vi "Json_Data_Path.vi"(8 "error in":errorcluster, 10 "ERD Data In":cluster{"ERD Number":u16, "Data":string}[](array[cluster]) {"ERD Number" format="%.0x"}, 11 "Json File Path":path) -> (0 "error out":errorcluster, 2 "ERD Data Out":cluster{"ERD Number":u16, "Data":string}[](array[cluster]) {"ERD Number" format="%.0x"})   [LabVIEW 2021]
uses:
  <vilib>/JDP Science/JSONtext/String Subset.vi
  <vilib>/JDP Science/JSONtext/support/Strip Quotes and Unescape.vi
  <vilib>/JDP Science/JSONtext/support/Unescape JSON string.vi
  <vilib>/JDP Science/JSONtext/Parsing/Parse Full Path or Item Name.vi
  <vilib>/JDP Science/JSONtext/Offset/Find Item Locations by Path.vi
  <vilib>/JDP Science/JSONtext/JSONtext.lvlib
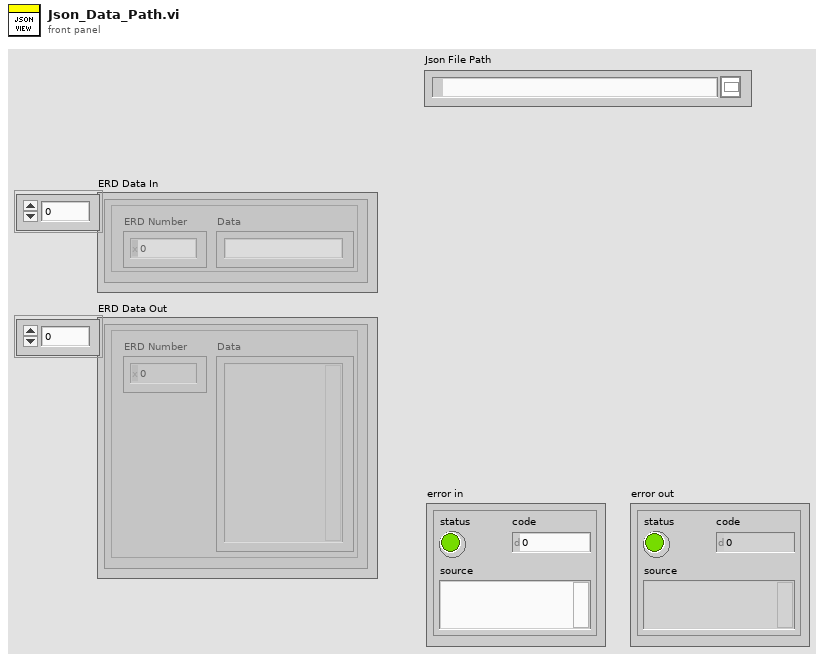
[diagram p1: front panel]
types:
  T1 = cluster{"ERD Data In[0]":cluster{"ERD Number":u16, "Data":string}, "ERD Data In[1]":cluster{"ERD Number":u16, "Data":string}, "ERD Data In[2]":cluster{"ERD Number":u16, "Data":string}, "ERD Data In[3]":cluster{"ERD Number":u16, "Data":string}, "ERD Data In[4]":cluster{"ERD Number":u16, "Data":string}, "ERD Data In[5]":cluster{"ERD Number":u16, "Data":string}, "ERD Data In[6]":cluster{"ERD Number":u16, "Data":string}, "ERD Data In[7]":cluster{"ERD Number":u16, "Data":string}, "ERD Data In[8]":cluster{"ERD Number":u16, "Data":string}}
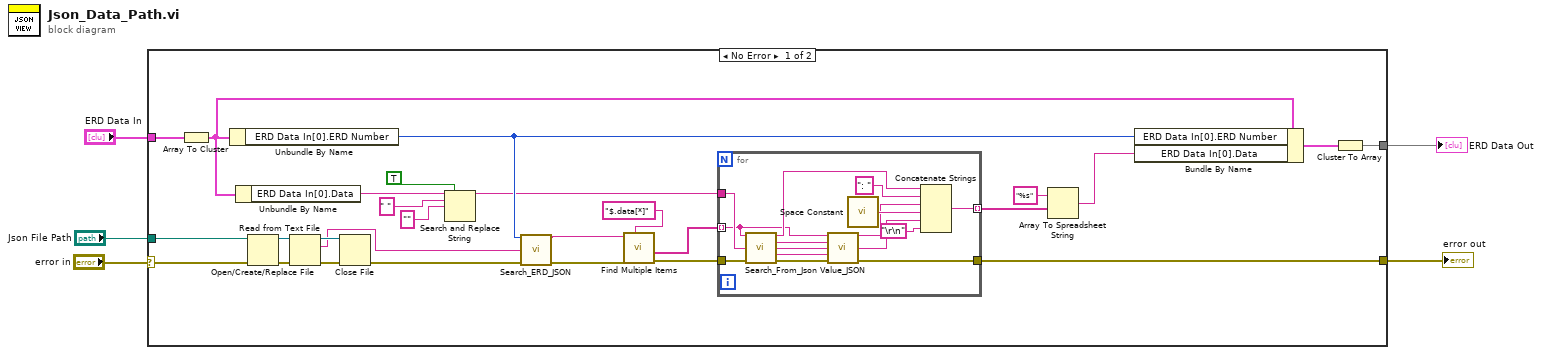
[diagram p0: block diagram]
diagram:
  n1 = case shown="No Error" "error in" {
    selector: "error in" -> [w16 w48]
    tunnel: [w7 w48] -> w4
    tunnel: "Json File Path" -> [w28 _]
    tunnel: "ERD Data In" -> [w27 _]
    tunnel: [w26 _] -> w1
    frame No Error {
      n2 = Array To Cluster(array=w27) -> (cluster=w6:T1)
      n3 = Unbundle By Name(w6) -> ("ERD Data In[0].ERD Number"=w12:u16)
      n4 = Unbundle By Name(w6) -> ("ERD Data In[0].Data"=w20:string)
      n5 = Open/Create/Replace File(file path (use dialog)=w28, error in=w16) -> (refnum out=w30:refnum<file>, error out=w32:errorcluster)  [unwired: 4 in, 1 out]
      n6 = Read from Text File(file (use dialog)=w30, error in=w32) -> (refnum out=w29:refnum<file>, text=w9:string, error out=w31:errorcluster)  [unwired: 2 in, 1 out]
      n7 = Close File(refnum=w29, error in=w31) -> (error out=w10:errorcluster)  [unwired: 1 out]
      n8 = Search and Replace String(replace all?=TRUE ("replace all? (F)"), input string=w20, search string=" ", replace string="" ("replace string (\"\")")) -> (result string=w8:string)  [unwired: 4 in, 3 out]
      n9 = call "Search_ERD_JSON.vi"("ERD Number"=w12, "JSON Text"=w9, "error in"=w10) -> ("ERD"=w13:string, "error out"=w14:errorcluster)  [unwired: 11 in]
      n10 = call <vilib>:"Find Multiple Items.vi"("$Path or Item Name"="$.data[*]", "error in (no error)"=w14, "JSON"=w13) -> ("error out"=w11:errorcluster, "<JSON>"=w24:string[])  [unwired: 5 in, 2 out]
      n11 = for {
        tunnel: w24 -> [w41] mode=indexing
        tunnel: w8 -> [w43]
        tunnel: [w45] -> w18 mode=indexing
        tunnel: [w34] -> w7
        tunnel: w11 -> [w33]
        n12 = call "Search_From_Json.vi"("Data JSON"=w41, "ERD"=w43, "error in"=w33) -> ("Name"=w42:string, "Type"=w40:string, "Size data"=w39:string, "Hexa"=w38:string, "error IO"=w37:errorcluster)  [unwired: 8 in]
        n13 = call "Value_JSON.vi"("Data JSON"=w41, "Type"=w40, "Size data"=w39, "Hexa"=w38, "error in"=w37) -> ("Value_string"=w36:string, "Hexa value"=w35:string, "error IO"=w34:errorcluster)  [unwired: 8 in]
        n14 = call <vilib>:"Space Constant.vi"() -> ("String"=w46:string)
        n15 = Concatenate Strings(w42, ": " ("string"), w36, w46, w35, "\r\n") -> (w45:string)
      }
      n16 = Array To Spreadsheet String(array=w18, 3:"%s" ("format string")) -> (spreadsheet string=w17:string)  [unwired: 1 in]
      n17 = Bundle By Name(cluster=w6, "ERD Data In[0].ERD Number"=w12, "ERD Data In[0].Data"=w17) -> (w15:T1)
      n18 = Cluster To Array(cluster=w15) -> (array=w26:cluster{"ERD Number":u16, "Data":string}[])
    }
    frame Error {
    }
  }
  "error out" <- w4
  "ERD Data Out" <- w1
